vi "New ListSelection.vi"(8 "error in (no error)":errorcluster, 10 "Bool Refnum":refnum<vi>, 11 "ListSelection in":refnum<class "ListSelection.lvclass">) -> (0 "error out":errorcluster, 3 "ListSelection out":refnum<class "ListSelection.lvclass">)   [LabVIEW 2015, in "Admin_Actor.lvlib" / "ListSelection.lvclass"]
uses:
  ListSelection.lvclass
  ListSelection.lvclass/ListSelection.ctl
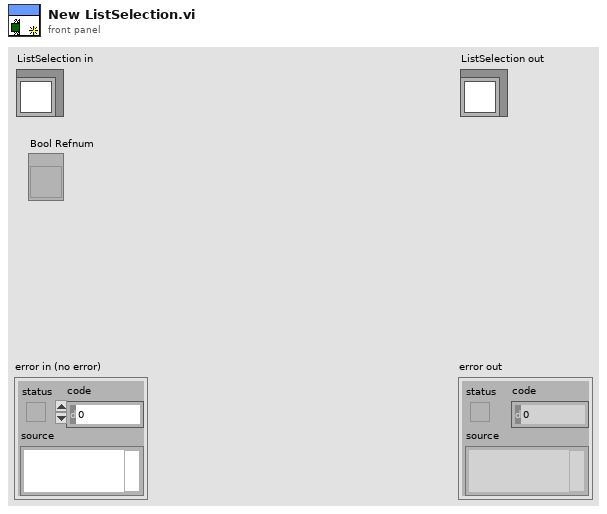
[diagram p1: front panel]
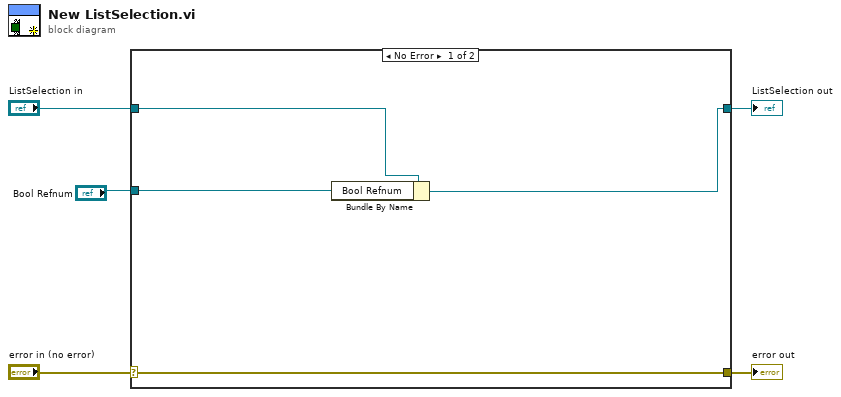
[diagram p0: block diagram]
diagram:
  n1 = case shown="No Error" "error in (no error)" {
    selector: "error in (no error)" -> [w9 w11]
    tunnel: [w9 w11] -> w4
    tunnel: [w7 w10] -> w2
    tunnel: "ListSelection in" -> [w8 w10]
    tunnel: "Bool Refnum" -> [w6 _]
    frame No Error {
      n2 = Bundle By Name(cluster=w8, "Bool Refnum"=w6) -> (w7:refnum<class "ListSelection.lvclass">)
    }
    frame Error {
    }
  }
  "error out" <- w4
  "ListSelection out" <- w2
